vi "Wait_Buf.vi"(5 "ReadParsIn":T3, 6 "ViStatusIn":T2, 7 "InterfaceInfoIn":T1, 8 "reference":refnum<vi>) -> (1 "ViStatusOut":T2, 2 "ReadPars":T3, 3 "InterfaceInfoOut":T1)   [LabVIEW 2010]
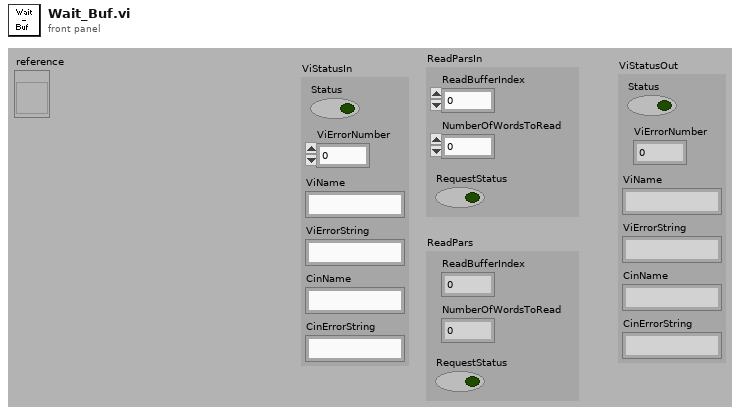
[diagram p1: front panel]
types:
  T1 = cluster{"DllVersion":u32, "InterfaceType":u32, "InterfaceInstance":u32, "ModuleHandle":u32, "ReadBuffersParsArray":cluster{"Buffer":i16[], "ReadOv":u32, "ReadEvent":u32}[], "WriteBuffersParsArray":cluster{"Buffer":i16[], "WriteOv":u32, "WriteEvent":u32}[]}
  T2 = cluster{"Status":bool, "ViErrorNumber":u32, "ViName":string, "ViErrorString":string, "CinName":string, "CinErrorString":string}
  T3 = cluster{"ReadBufferIndex":u32, "NumberOfWordsToRead":u32, "RequestStatus":bool}
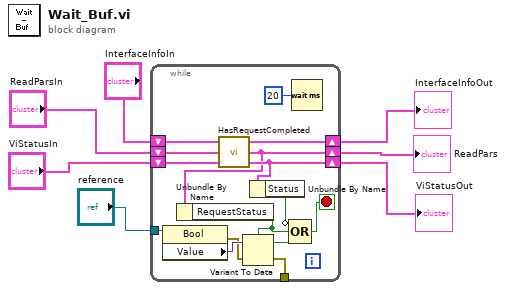
[diagram p0: block diagram]
diagram:
  n1 = while {
    shift-right: [w9] -> w7
    shift-left: "InterfaceInfoIn" -> [w14]
    shift-right: [w10] -> w6
    shift-left: "ReadParsIn" -> [w13]
    shift-right: [w11] -> w4
    shift-left: "ViStatusIn" -> [w12]
    tunnel: "reference" -> [w20]
    tunnel: [w8] -> _
    stop <- w22 stop-if-true
    n2 = property class="Bool"(reference=w20) -> (error out=w17:errorcluster, "Value"=w18:variant)  [unwired: 1 in, 1 out]
    n3 = call "HasRequestCompleted.vi"("ViStatusIn"=w12, "ReadParsIn"=w13, "InterfaceInfoIn"=w14) -> ("ViStatusOut"=w11:T2, "ReadParsOut"=w10:T3, "InterfaceInfoOut"=w9:T1)
    n4 = Unbundle By Name(w10) -> ("RequestStatus"=w16:bool)
    n5 = Variant To Data(error in=w17, Variant=w18, type=w16) -> (error out=w8:errorcluster, data=w15:bool)
    n6 = Unbundle By Name(w11) -> ("Status"=w21:bool)
    n7 = Compound Arithmetic op=OR(invert w21, w16, w15) -> (w22:bool)
    n8 = Wait (ms)(milliseconds to wait=u32 20) -> ()  [unwired: 1 out]
  }
  "InterfaceInfoOut" <- w7
  "ReadPars" <- w6
  "ViStatusOut" <- w4
